vi "Autonomous Independent.vi"() -> ()   [LabVIEW 2016]
doc: "This VI is called when autonomous begins, and will automatically be terminated when autonomous ends. You can carry out timed or sensor driven robot movement independently without needing to return to the caller."
uses:
  <vilib>/Rock Robotics/Network Tables/NT Read Number.vi
  Global 2.vi
  Systems/Global 1.vi
panel:
  out "Waveform Graph":dbl[](graph)=[24.733139233474137]
  out "Numeric":i32=72
  out "Gyro":dbl=0.0502646432904
  in  "Oscillate effort":dbl=0.25 format="%#_13g"
  out "Auto Mode":dbl=2.0
  in  "Auton_Modes":T1(array[cluster])=[{"Actions"=[{"Effort"=0.55, "Duration"=3.5, "Action"=enum."Vision Correction", "Encoder"=0.0, "Condition"=FALSE}, {"Effort"=0.0, "Duration"=0.0, "Action"=enum."Nothing", "Encoder"=0.0, "Condition"=FALSE}]}, {"Actions"=[{"Effort"=0.53, "Duration"=1.0, "Action"=enum."Shoot", "Encoder"=6.462, "Condition"=TRUE}, {"Effort"=0.0, "Duration"=3.0, "Action"=enum."Index", "Encoder"=0.0, "Condition"=FALSE}, {"Effort"=0.3, "Duration"=2.0, "Action"=enum."Turn", "Encoder"=38.0, "Condition"=FALSE}, {"Effort"=0.3, "Duration"=5.0, "Action"=enum."Drive", "Encoder"=0.0, "Condition"=TRUE}, {"Effort"=0.25, "Duration"=0.0, "Action"=enum."Nothing", "Encoder"=57.0, "Condition"=FALSE}, {"Effort"=-0.25, "Duration"=0.0, "Action"=enum."Nothing", "Encoder"=0.0, "Condition"=FALSE}, {"Effort"=1.0, "Duration"=0.0, "Action"=enum."Nothing", "Encoder"=0.0, "Condition"=FALSE}, {"Effort"=0.25, "Duration"=0.0, "Action"=enum."Nothing", "Encoder"=0.0, "Condition"=FALSE}]}, {"Actions"=[{"Effort"=0.0, "Duration"=0.1, "Action"=enum."Drive Encoder Reset", "Encoder"=0.0, "Condition"=FALSE}, {"Effort"=0.0, "Duration"=0.1, "Action"=enum."Gyro Reset", "Encoder"=0.0, "Condition"=FALSE}, {"Effort"=0.3, "Duration"=2.5, "Action"=enum."Drive", "Encoder"=50.0, "Condition"=FALSE}, {"Effort"=1.0, "Duration"=1.0, "Action"=enum."Gear0", "Encoder"=0.0, "Condition"=FALSE}, {"Effort"=1.0, "Duration"=0.0, "Action"=enum."Nothing", "Encoder"=0.0, "Condition"=FALSE}, {"Effort"=1.0, "Duration"=0.5, "Action"=enum."Nothing", "Encoder"=0.0, "Condition"=FALSE}, {"Effort"=0.0, "Duration"=0.0, "Action"=enum."Drive Encoder Reset", "Encoder"=0.0, "Condition"=FALSE}, {"Effort"=0.3, "Duration"=0.5, "Action"=enum."Nothing", "Encoder"=10.0, "Condition"=FALSE}, {"Effort"=0.0, "Duration"=0.0, "Action"=enum."Nothing", "Encoder"=0.0, "Condition"=FALSE}, {"Effort"=-0.2, "Duration"=10000.0, "Action"=enum."Drive", "Encoder"=24.0, "Condition"=FALSE}, {"Effort"=0.0, "Duration"=0.0, "Action"=enum."Drive Encoder Reset", "Encoder"=0.0, "Condition"=FALSE}, {"Effort"=-0.25, "Duration"=0.0, "Action"=enum."Nothing", "Encoder"=12.0, "Condition"=FALSE}]}, {"Actions"=[{"Effort"=0.0, "Duration"=0.1, "Action"=enum."Drive Encoder Reset", "Encoder"=6.462, "Condition"=FALSE}, {"Effort"=0.0, "Duration"=0.1, "Action"=enum."Gyro Reset", "Encoder"=0.0, "Condition"=FALSE}, {"Effort"=-0.25, "Duration"=1.0, "Action"=enum."Drive", "Encoder"=6.462, "Condition"=FALSE}, {"Effort"=0.0, "Duration"=0.1, "Action"=enum."Gyro Reset", "Encoder"=0.0, "Condition"=FALSE}, {"Effort"=-0.25, "Duration"=0.0, "Action"=enum."Turn", "Encoder"=0.0, "Condition"=FALSE}, {"Effort"=-0.25, "Duration"=0.0, "Action"=enum."Drive", "Encoder"=7.5, "Condition"=FALSE}, {"Effort"=-1.0, "Duration"=0.0, "Action"=enum."Gear0", "Encoder"=0.0, "Condition"=FALSE}, {"Effort"=0.25, "Duration"=0.0, "Action"=enum."Drive", "Encoder"=3.0, "Condition"=FALSE}]}, {"Actions"=[{"Effort"=0.0, "Duration"=0.1, "Action"=enum."Drive Encoder Reset", "Encoder"=6.462, "Condition"=FALSE}, {"Effort"=0.0, "Duration"=0.1, "Action"=enum."Gyro Reset", "Encoder"=0.0, "Condition"=FALSE}, {"Effort"=-0.25, "Duration"=1.0, "Action"=enum."Drive", "Encoder"=6.462, "Condition"=FALSE}, {"Effort"=0.0, "Duration"=0.1, "Action"=enum."Gyro Reset", "Encoder"=0.0, "Condition"=FALSE}, {"Effort"=-0.25, "Duration"=0.0, "Action"=enum."Turn", "Encoder"=0.0, "Condition"=FALSE}, {"Effort"=-0.25, "Duration"=0.0, "Action"=enum."Drive", "Encoder"=7.5, "Condition"=FALSE}, {"Effort"=-1.0, "Duration"=0.0, "Action"=enum."Gear0", "Encoder"=0.0, "Condition"=FALSE}, {"Effort"=0.25, "Duration"=0.0, "Action"=enum."Drive", "Encoder"=3.0, "Condition"=FALSE}]}, {"Actions"=[{"Effort"=0.0, "Duration"=0.1, "Action"=enum."Drive Encoder Reset", "Encoder"=0.0, "Condition"=FALSE}, {"Effort"=0.0, "Duration"=0.1, "Action"=enum."Gyro Reset", "Encoder"=0.0, "Condition"=FALSE}, {"Effort"=0.25, "Duration"=1.0, "Action"=enum."Drive", "Encoder"=6.462, "Condition"=FALSE}, {"Effort"=1.0, "Duration"=0.1, "Action"=enum."Gyro Reset", "Encoder"=0.0, "Condition"=FALSE}, {"Effort"=0.25, "Duration"=0.0, "Action"=enum."Turn", "Encoder"=0.0, "Condition"=FALSE}, {"Effort"=0.25, "Duration"=0.0, "Action"=enum."Drive", "Encoder"=7.5, "Condition"=FALSE}, {"Effort"=1.0, "Duration"=0.0, "Action"=enum."Gear0", "Encoder"=0.0, "Condition"=FALSE}, {"Effort"=-0.25, "Duration"=0.0, "Action"=enum."Drive", "Encoder"=3.0, "Condition"=FALSE}]}, {"Actions"=[{"Effort"=0.0, "Duration"=0.1, "Action"=enum."Nothing", "Encoder"=0.0, "Condition"=FALSE}, {"Effort"=0.0, "Duration"=0.1, "Action"=enum."Gyro Reset", "Encoder"=0.0, "Condition"=FALSE}, {"Effort"=0.25, "Duration"=5.0, "Action"=enum."Drive", "Encoder"=60000.0, "Condition"=TRUE}, {"Effort"=0.75, "Duration"=1.0, "Action"=enum."Nothing", "Encoder"=0.0, "Condition"=FALSE}, {"Effort"=0.0, "Duration"=1.0, "Action"=enum."Nothing", "Encoder"=0.0, "Condition"=FALSE}, {"Effort"=0.0, "Duration"=0.0, "Action"=enum."Nothing", "Encoder"=0.0, "Condition"=FALSE}]}, {"Actions"=[{"Effort"=0.0, "Duration"=0.5, "Action"=enum."Drive Encoder Reset", "Encoder"=0.0, "Condition"=FALSE}, {"Effort"=0.55, "Duration"=4.25, "Action"=enum."Gyro Reset", "Encoder"=0.0, "Condition"=FALSE}, {"Effort"=-0.5, "Duration"=0.0, "Action"=enum."Drive", "Encoder"=46.0, "Condition"=FALSE}, {"Effort"=0.3, "Duration"=1.0, "Action"=enum."Nothing", "Encoder"=0.0, "Condition"=FALSE}, {"Effort"=0.3, "Duration"=2.0, "Action"=enum."Vision Correction", "Encoder"=76.6, "Condition"=FALSE}, {"Effort"=-0.25, "Duration"=1.0, "Action"=enum."Drive", "Encoder"=18.5, "Condition"=TRUE}, {"Effort"=1.0, "Duration"=0.0, "Action"=enum."Gear0", "Encoder"=0.0, "Condition"=FALSE}, {"Effort"=0.3, "Duration"=1.3, "Action"=enum."Drive", "Encoder"=30.0, "Condition"=TRUE}, {"Effort"=0.0, "Duration"=0.0, "Action"=enum."Nothing", "Encoder"=0.0, "Condition"=FALSE}, {"Effort"=0.03, "Duration"=0.0, "Action"=enum."Turn", "Encoder"=0.0, "Condition"=FALSE}, {"Effort"=0.0, "Duration"=0.0, "Action"=enum."Drive", "Encoder"=0.0, "Condition"=FALSE}]}, {"Actions"=[{"Effort"=0.0, "Duration"=0.0, "Action"=enum."Nothing", "Encoder"=0.0, "Condition"=FALSE}]}, {"Actions"=[{"Effort"=0.0, "Duration"=2.5, "Action"=enum."Shoot", "Encoder"=0.0, "Condition"=FALSE}, {"Effort"=0.0, "Duration"=5.0, "Action"=enum."Index", "Encoder"=0.0, "Condition"=FALSE}, {"Effort"=0.25, "Duration"=3.5, "Action"=enum."Nothing", "Encoder"=88.0, "Condition"=FALSE}, {"Effort"=1.0, "Duration"=1.0, "Action"=enum."Nothing", "Encoder"=0.0, "Condition"=FALSE}, {"Effort"=1.0, "Duration"=1.0, "Action"=enum."Nothing", "Encoder"=0.0, "Condition"=FALSE}, {"Effort"=1.0, "Duration"=0.5, "Action"=enum."Nothing", "Encoder"=0.0, "Condition"=FALSE}, {"Effort"=0.0, "Duration"=0.0, "Action"=enum."Nothing", "Encoder"=0.0, "Condition"=FALSE}, {"Effort"=-0.25, "Duration"=0.0, "Action"=enum."Nothing", "Encoder"=3.0, "Condition"=FALSE}, {"Effort"=0.0, "Duration"=0.0, "Action"=enum."Nothing", "Encoder"=0.0, "Condition"=FALSE}, {"Effort"=0.25, "Duration"=0.0, "Action"=enum."Nothing", "Encoder"=24.0, "Condition"=FALSE}, {"Effort"=0.0, "Duration"=0.0, "Action"=enum."Nothing", "Encoder"=0.0, "Condition"=FALSE}, {"Effort"=-0.25, "Duration"=0.0, "Action"=enum."Nothing", "Encoder"=12.0, "Condition"=FALSE}]}, {"Actions"=[{"Effort"=0.0, "Duration"=0.1, "Action"=enum."Drive Encoder Reset", "Encoder"=0.0, "Condition"=FALSE}, {"Effort"=0.0, "Duration"=1.0, "Action"=enum."Gyro Reset", "Encoder"=0.0, "Condition"=FALSE}, {"Effort"=0.3, "Duration"=1.4, "Action"=enum."Drive", "Encoder"=88.0, "Condition"=TRUE}, {"Effort"=0.3, "Duration"=4.0, "Action"=enum."Turn", "Encoder"=2.0, "Condition"=FALSE}, {"Effort"=1.0, "Duration"=1.0, "Action"=enum."Nothing", "Encoder"=0.0, "Condition"=FALSE}, {"Effort"=1.0, "Duration"=0.5, "Action"=enum."Nothing", "Encoder"=0.0, "Condition"=FALSE}, {"Effort"=0.0, "Duration"=0.0, "Action"=enum."Nothing", "Encoder"=0.0, "Condition"=FALSE}, {"Effort"=-0.25, "Duration"=0.0, "Action"=enum."Nothing", "Encoder"=3.0, "Condition"=FALSE}, {"Effort"=0.0, "Duration"=0.0, "Action"=enum."Nothing", "Encoder"=0.0, "Condition"=FALSE}, {"Effort"=0.25, "Duration"=0.0, "Action"=enum."Nothing", "Encoder"=24.0, "Condition"=FALSE}, {"Effort"=0.0, "Duration"=0.0, "Action"=enum."Nothing", "Encoder"=0.0, "Condition"=FALSE}, {"Effort"=-0.25, "Duration"=0.0, "Action"=enum."Nothing", "Encoder"=12.0, "Condition"=FALSE}]}, {"Actions"=[{"Effort"=0.0, "Duration"=1.0, "Action"=enum."Drive Encoder Reset", "Encoder"=0.0, "Condition"=FALSE}, {"Effort"=0.0, "Duration"=1.0, "Action"=enum."Shoot", "Encoder"=0.0, "Condition"=FALSE}, {"Effort"=0.25, "Duration"=5.0, "Action"=enum."Index", "Encoder"=88.0, "Condition"=FALSE}, {"Effort"=1.0, "Duration"=1.0, "Action"=enum."Nothing", "Encoder"=0.0, "Condition"=FALSE}, {"Effort"=1.0, "Duration"=1.0, "Action"=enum."Nothing", "Encoder"=0.0, "Condition"=FALSE}, {"Effort"=1.0, "Duration"=0.5, "Action"=enum."Nothing", "Encoder"=0.0, "Condition"=FALSE}, {"Effort"=0.0, "Duration"=0.0, "Action"=enum."Nothing", "Encoder"=0.0, "Condition"=FALSE}, {"Effort"=-0.25, "Duration"=0.0, "Action"=enum."Nothing", "Encoder"=3.0, "Condition"=FALSE}, {"Effort"=0.0, "Duration"=0.0, "Action"=enum."Nothing", "Encoder"=0.0, "Condition"=FALSE}, {"Effort"=0.25, "Duration"=0.0, "Action"=enum."Nothing", "Encoder"=24.0, "Condition"=FALSE}, {"Effort"=0.0, "Duration"=0.0, "Action"=enum."Nothing", "Encoder"=0.0, "Condition"=FALSE}, {"Effort"=-0.25, "Duration"=0.0, "Action"=enum."Nothing", "Encoder"=12.0, "Condition"=FALSE}]}, {"Actions"=[{"Effort"=0.0, "Duration"=0.1, "Action"=enum."Drive Encoder Reset", "Encoder"=0.0, "Condition"=FALSE}, {"Effort"=0.0, "Duration"=1.0, "Action"=enum."Gyro Reset", "Encoder"=0.0, "Condition"=FALSE}, {"Effort"=0.3, "Duration"=1.4, "Action"=enum."Drive", "Encoder"=88.0, "Condition"=TRUE}, {"Effort"=0.3, "Duration"=4.0, "Action"=enum."Turn", "Encoder"=0.0, "Condition"=FALSE}, {"Effort"=1.0, "Duration"=1.0, "Action"=enum."Nothing", "Encoder"=0.0, "Condition"=FALSE}, {"Effort"=1.0, "Duration"=0.5, "Action"=enum."Nothing", "Encoder"=0.0, "Condition"=FALSE}, {"Effort"=0.0, "Duration"=0.0, "Action"=enum."Nothing", "Encoder"=0.0, "Condition"=FALSE}, {"Effort"=0.3, "Duration"=0.5, "Action"=enum."Nothing", "Encoder"=24.0, "Condition"=TRUE}, {"Effort"=0.0, "Duration"=0.0, "Action"=enum."Nothing", "Encoder"=0.0, "Condition"=FALSE}, {"Effort"=-0.2, "Duration"=2.0, "Action"=enum."Nothing", "Encoder"=24.0, "Condition"=TRUE}, {"Effort"=0.0, "Duration"=0.0, "Action"=enum."Nothing", "Encoder"=0.0, "Condition"=FALSE}, {"Effort"=-0.25, "Duration"=0.0, "Action"=enum."Nothing", "Encoder"=12.0, "Condition"=FALSE}]}]
  # "Nothing"
  # "Boiler Right Right side gear"
  # "Middle Gear"
  # "Boiler Right Left Side Gear"
  # "Boiler Left RightSide Gear"
  # "Boiler Left Left Side Gear"
  # "Drive"
  # "Vision Correction"
  # "Hopper"
  # "10 ball"
  # "Farside"
  # "Boilerside-10 ball"
  # "Auto 5"
  # "Auto 6"
  # "Auto 6"
  # "Auto 7"
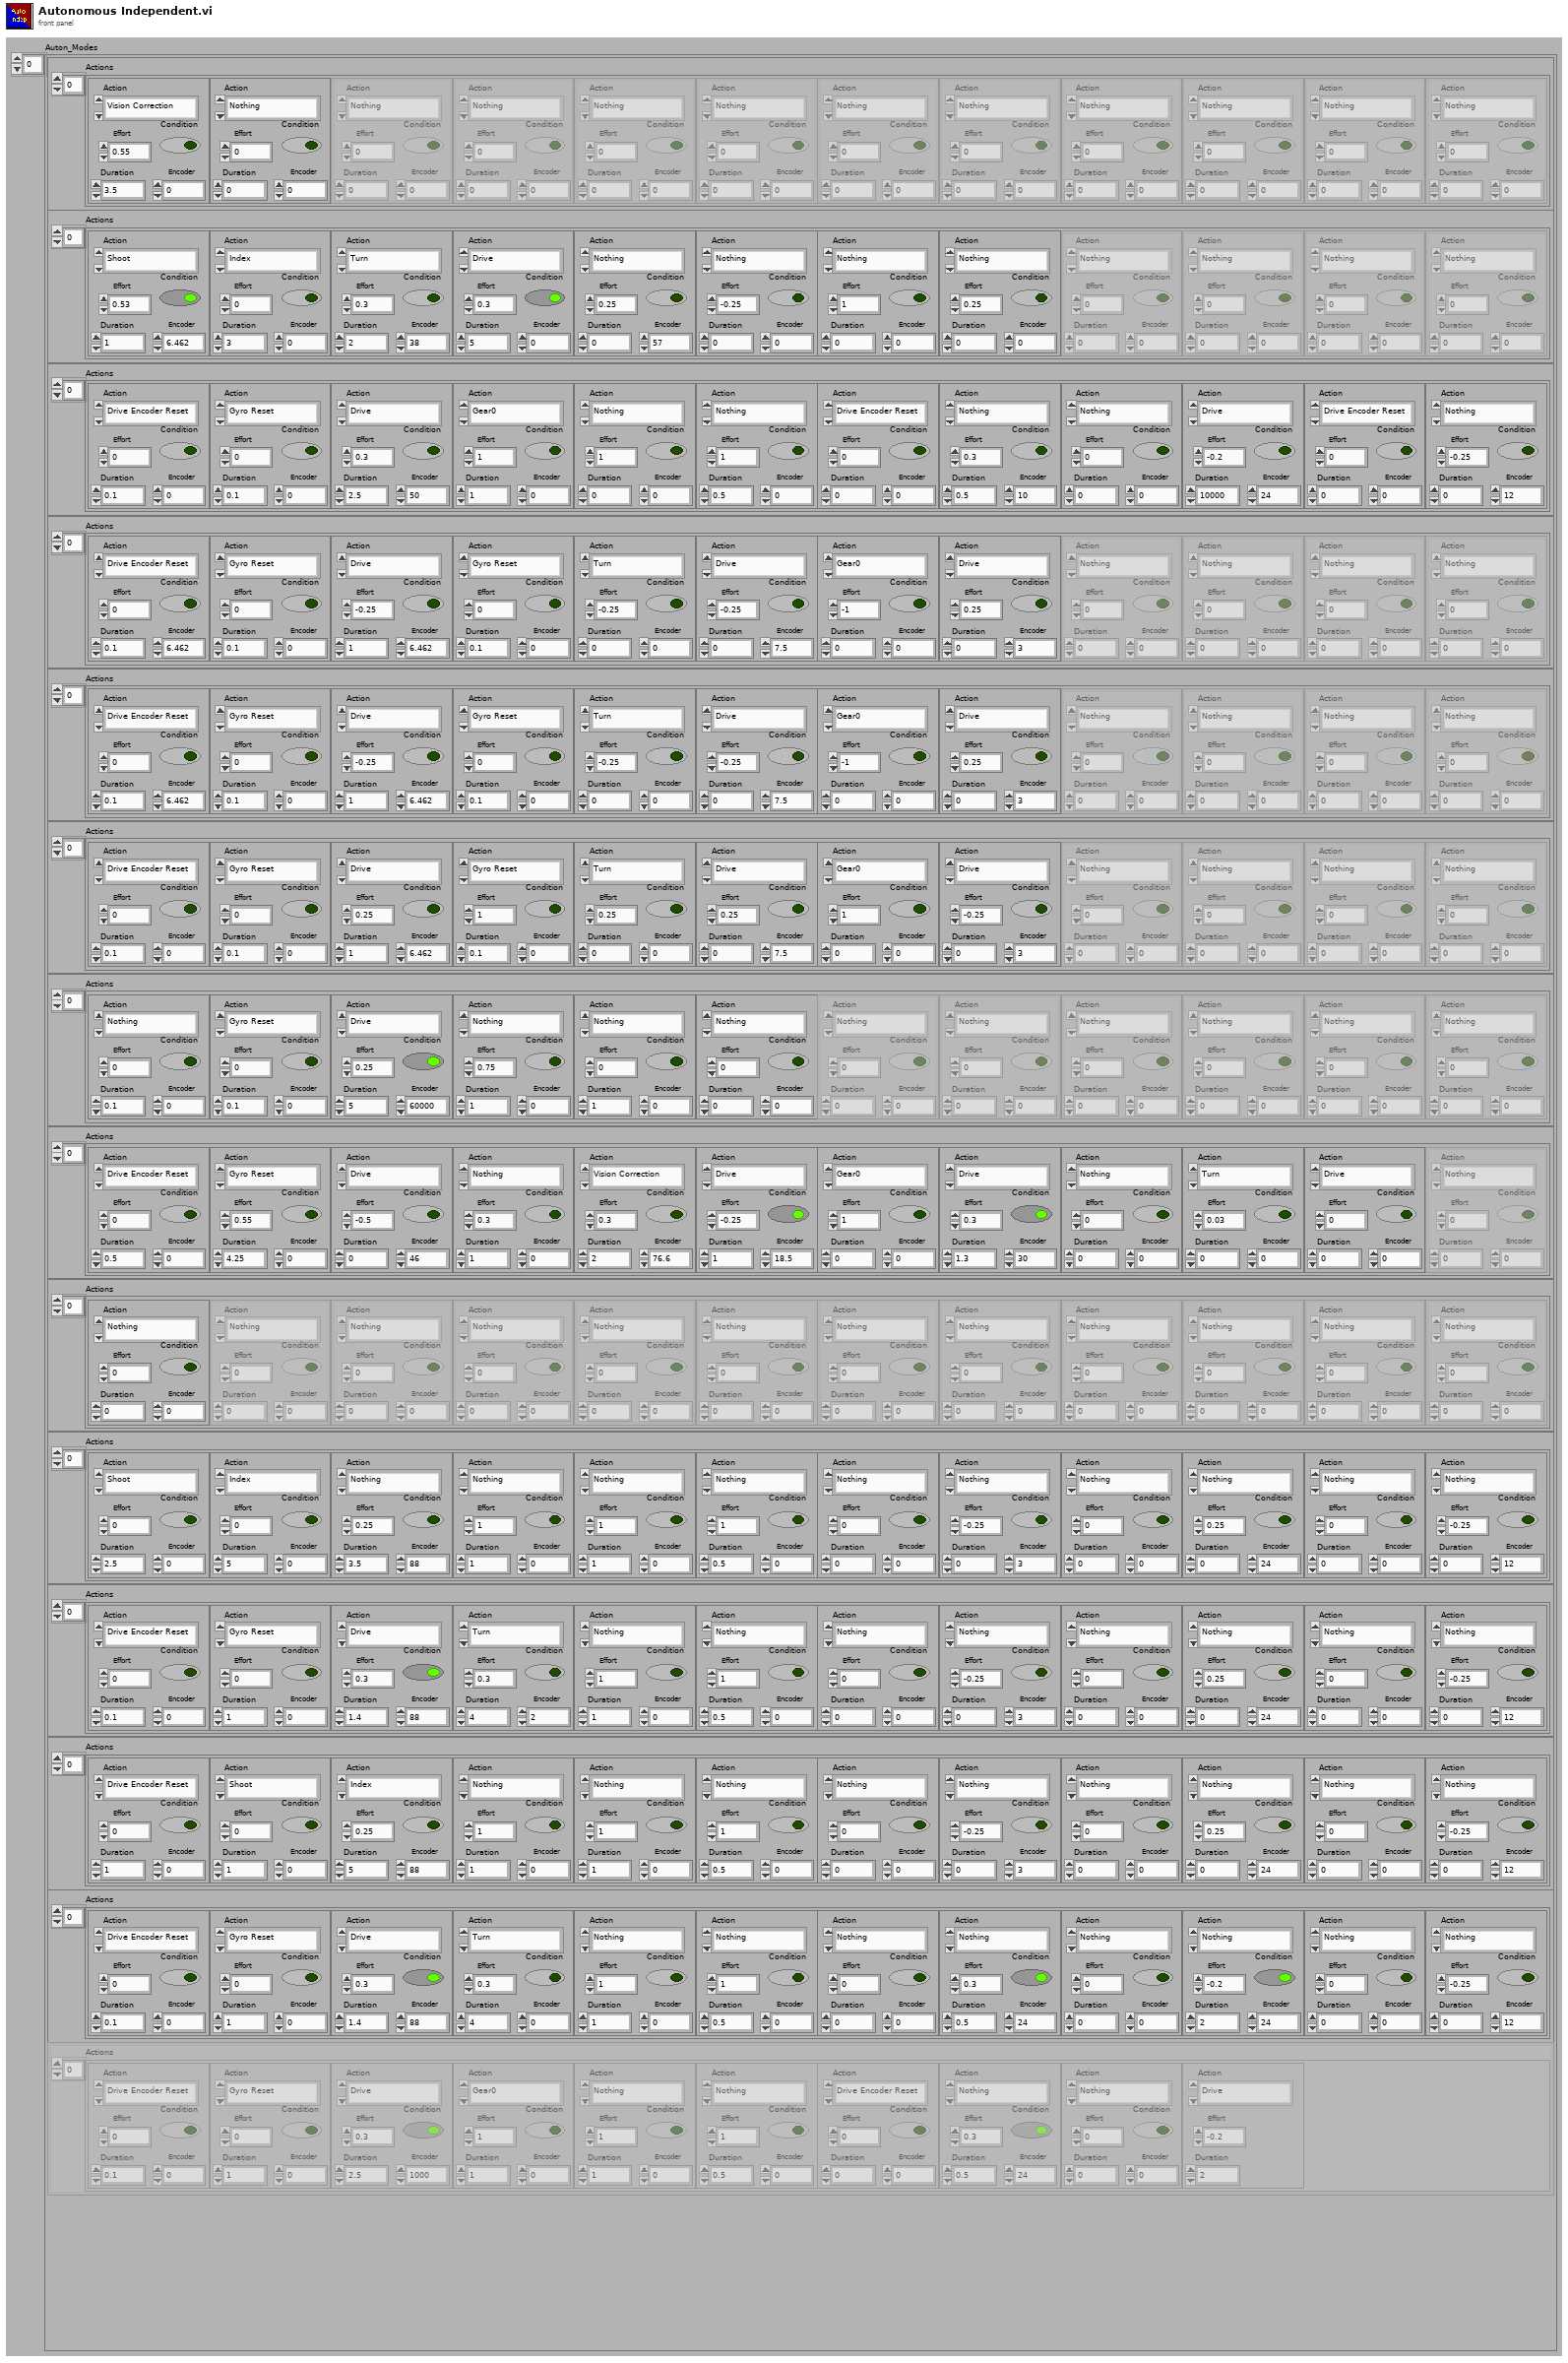
[diagram p1: front panel]
types:
  T1 = cluster{"Actions":cluster{"Effort":dbl, "Duration":dbl, "Action":enum16{"Nothing", "Drive", "Vision Correction", "Turn", "Gear0", "Gear1", "Climb", "Intake", "Index", "Shoot", "Test", "Drive Encoder Reset", "Gyro Reset"}, "Encoder":dbl, "Condition":bool}[]}[]
  T2 = cluster{"Actions":cluster{"Effort":dbl, "Duration":dbl, "Action":enum16{"Nothing", "Drive", "Vision Correction", "Turn", "Gear0", "Gear1", "Climb", "Intake", "Index", "Shoot", "Test", "Drive Encoder Reset", "Gyro Reset"}, "Encoder":dbl, "Condition":bool}[]}
  T3 = cluster{"Effort":dbl, "Duration":dbl, "Action":enum16{"Nothing", "Drive", "Vision Correction", "Turn", "Gear0", "Gear1", "Climb", "Intake", "Index", "Shoot", "Test", "Drive Encoder Reset", "Gyro Reset"}, "Encoder":dbl, "Condition":bool}[]
  T4 = enum16{"Nothing", "Drive", "Vision Correction", "Turn", "Gear0", "Gear1", "Climb", "Intake", "Index", "Shoot", "Test", "Drive Encoder Reset", "Gyro Reset"}
  T5 = typedef "WPI_MotorControlDeviceRef.ctl" = cluster{"DeviceStatus":errorcluster, "Type":T6, "PWM":cluster{"PWM Channel":T7, "DeadBand":T8}, "CAN":cluster{"Device Number":u8, "SetOutput VI Ref":variant, "GetOutput VI Ref":variant, "Enable VI Ref":variant, "Disable VI Ref":variant, "Data":variant}, "Invert":bool}
  T6 = typedef "WPI_MotorControlType.ctl" = enum16{"PWM", "CAN"}
  T7 = typedef "FPGA_DIOPWMChannel.ctl" = enum8{"PWM 0", "PWM 1", "PWM 2", "PWM 3", "PWM 4", "PWM 5", "PWM 6", "PWM 7", "PWM 8", "PWM 9", "PWM MXP 0", "PWM MXP 1", "PWM MXP 2", "PWM MXP 3", "PWM MXP 4", "PWM MXP 5", "PWM MXP 6", "PWM MXP 7", "PWM MXP 8", "PWM MXP 9", "Invalid"}
  T8 = typedef "WPI_PWMDeadband.ctl" = cluster{"Name":string, "maxPositivePwm":i32, "minPositivePwm":i32, "centerPwm":i32, "maxNegativePwm":i32, "minNegativePwm":i32, "angularRange":u16}
  T9 = typedef "WPI_CANTalonSRX_GlobalStatus.ctl" = cluster{"Applied Throttle":dbl, "Module Enabled":bool, "CAN Error":errorcluster, "Closed Loop Error":dbl, "Forward Limit Switch Closed":bool, "Reverse Limit Switch Closed":bool, "Sensor Position":dbl, "Sensor Velocity":dbl, "Current":dbl, "Sticky Fault - Over Temp":bool, "Sticky Fault - Under Voltage":bool, "Sticky Fault - Forward Limit":bool, "Sticky Fault - Reverse Limit":bool, "Sticky Fault - Forward Soft Limit":bool, "Sticky Fault - Reverse Soft Limit":bool, "Brake is Enabled":bool, "Encoder Position":dbl, "Encoder Velocity":dbl, "Encoder Index Count":dbl, "Encoder A Pin State":bool, "Encoder B Pin State":bool, "Encoder Index Pin State":bool, "Analog In":dbl, "Analog In Velocity":dbl, "Temperature (C)":dbl, "Battery Voltage":dbl, "Control 5 Is Supported":bool, "Current Profile Slot Select":dbl, "Pos Div 8":bool, "Vel Div 4":bool, "Pulse Width Position":i32, "Pulse Width Velocity":i32, "Pulse Width Rise To Rise (us)":i32, "Pulse Width Rise To Fall (us)":i32, "Mot Prof Active Is Under Run":bool, "Mot Prof Active Has Under Run":bool, "Mot Prof Active Is Last":bool, "Mot Prof Active Velocity Only":bool, "Mot Prof Active Is Valid":bool, "Mot Prof Buffer Is Full":bool, "Mot Prof Active Profile Slot Select":i32, "Mot Prof NextID":i32, "Mot Prof Count":i32, "Mot Prof Active Velocity":dbl, "Mot Prof Active Position":dbl, "Mot Prof Output Enable":i32}
  T10 = typedef "WPI_GyroDevRef.ctl" = cluster{"DevStatus":errorcluster, "Analog Channel":T11, "Offset":dbl, "Gain (VoltsPerDegree/Second)":dbl, "Gyro Type":enum16{"Analog", "XRS450"}, "Handle":i32, "SPI Bus":T12, "Device Found":bool, "Sample Rate":dbl, "Calibrate On Open":bool}
  T11 = typedef "FPGA_AIChannel.ctl" = enum8{"AI 0", "AI 1", "AI 2", "AI 3", "AI MXP 0", "AI MXP 1", "AI MXP 2", "AI MXP 3", "Invalid"}
  T12 = typedef "spi_bus.ctl" = enum16{"SPI On-Board, CS0", "SPI On-Board, CS1", "SPI On-Board, CS2", "SPI On-Board, CS3", "SPI MXP", "Invalid"}
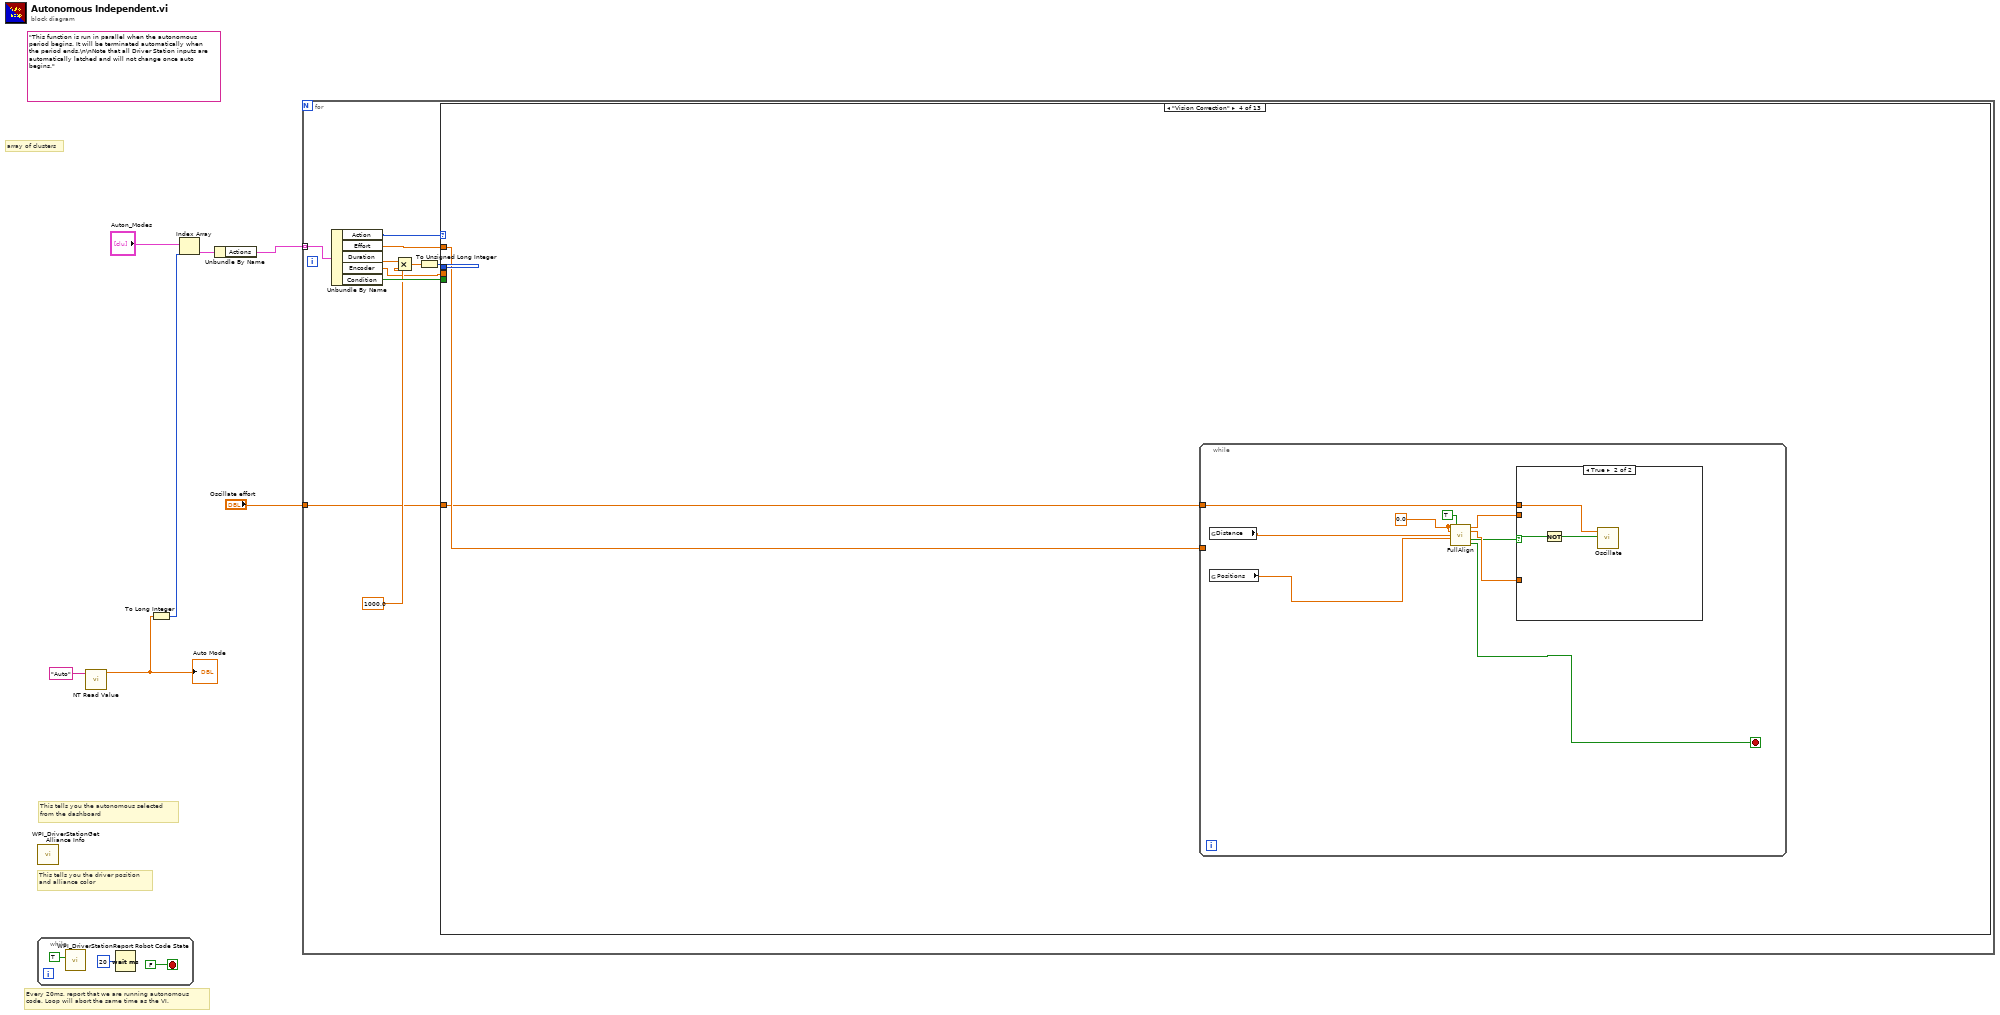
[diagram p0: block diagram]
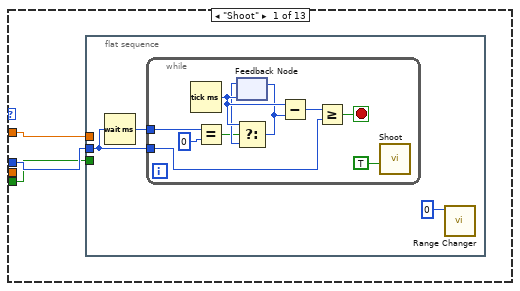
[diagram p2: hidden frame]
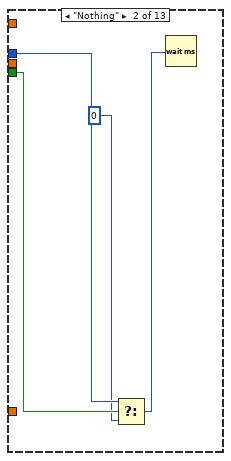
[diagram p3: hidden frame]
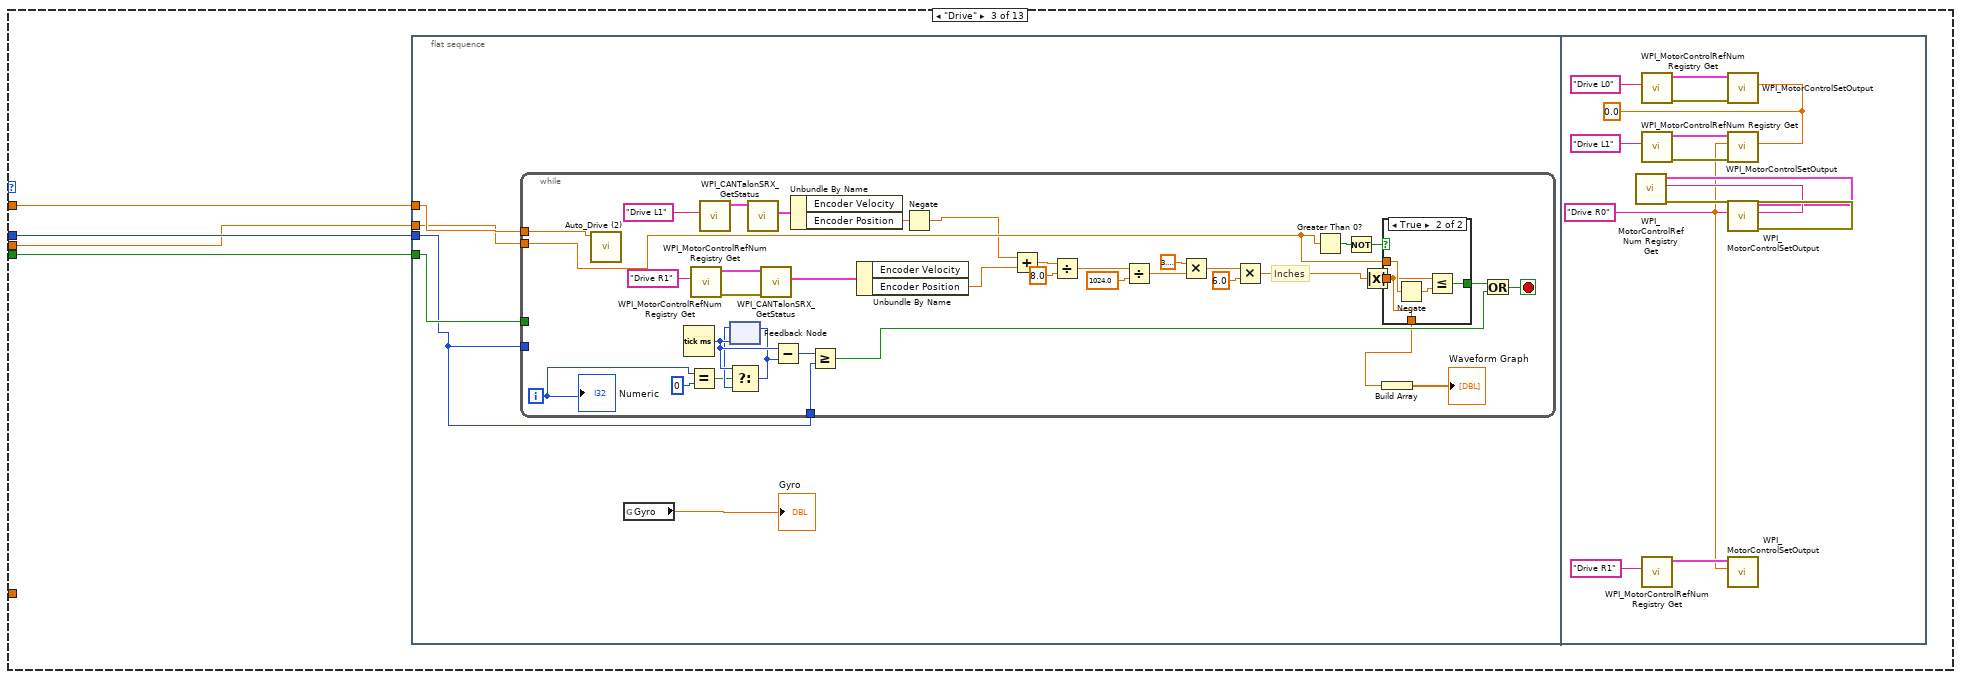
[diagram p4: hidden frame]
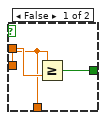
[diagram p5: hidden frame]
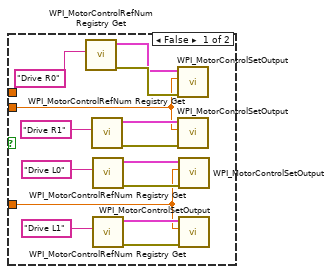
[diagram p6: hidden frame]
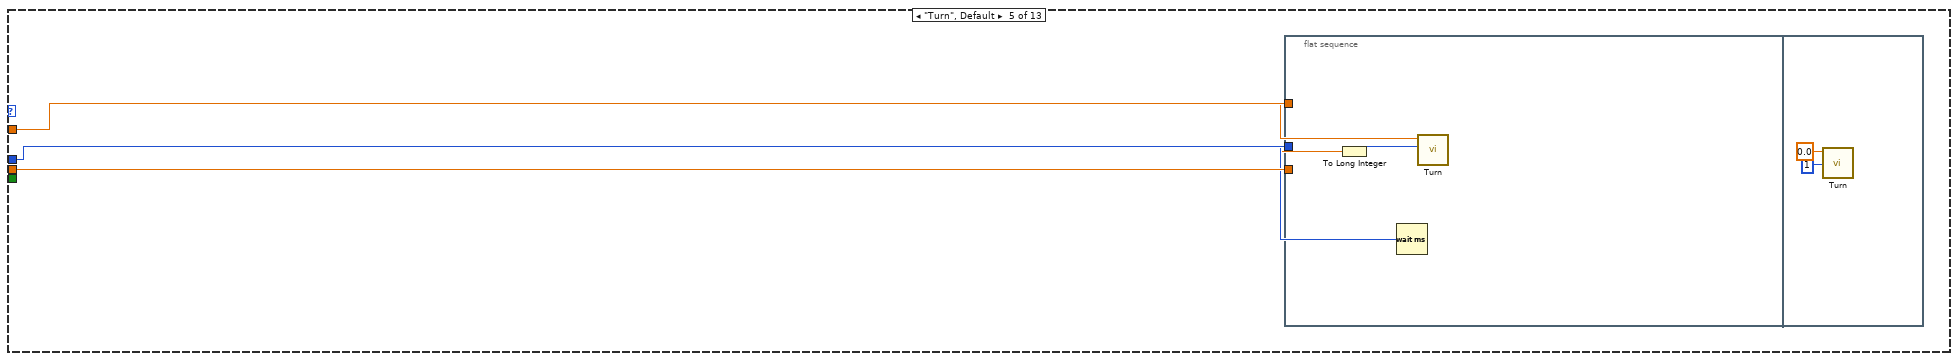
[diagram p7: hidden frame]
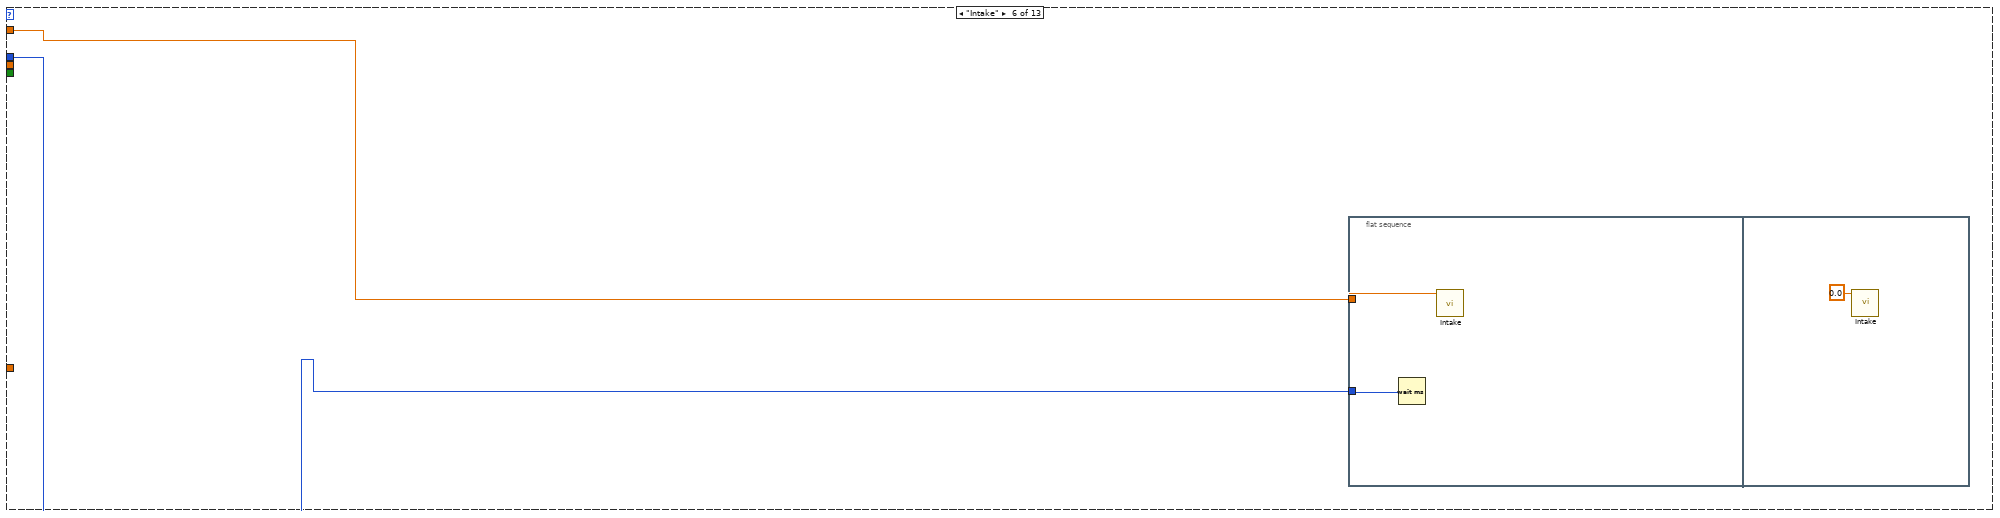
[diagram p8: hidden frame]
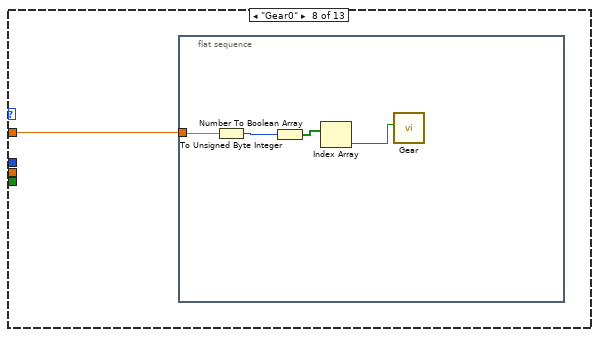
[diagram p10: hidden frame]
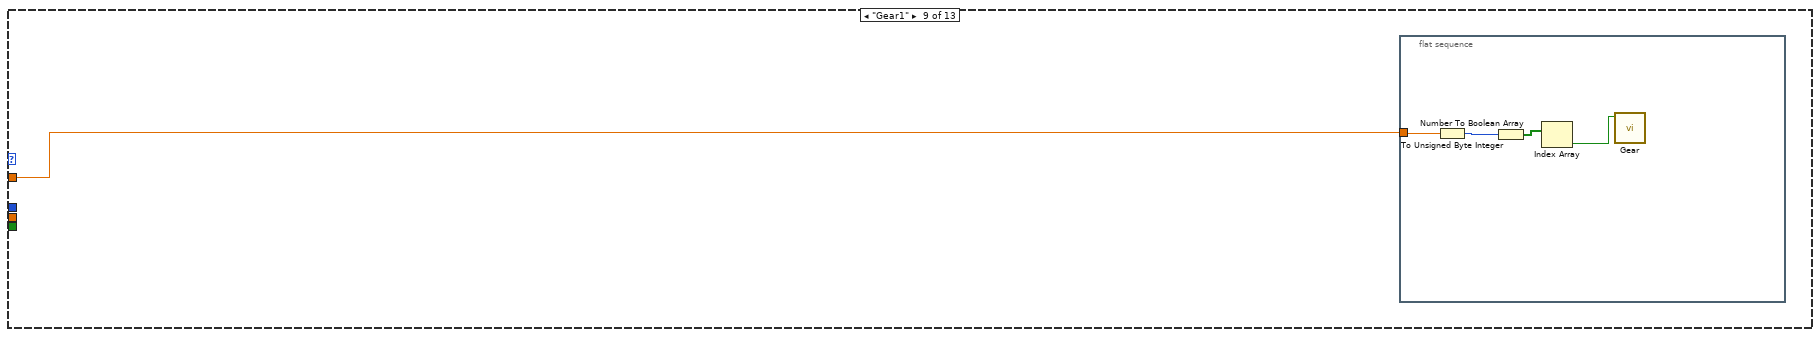
[diagram p11: hidden frame]
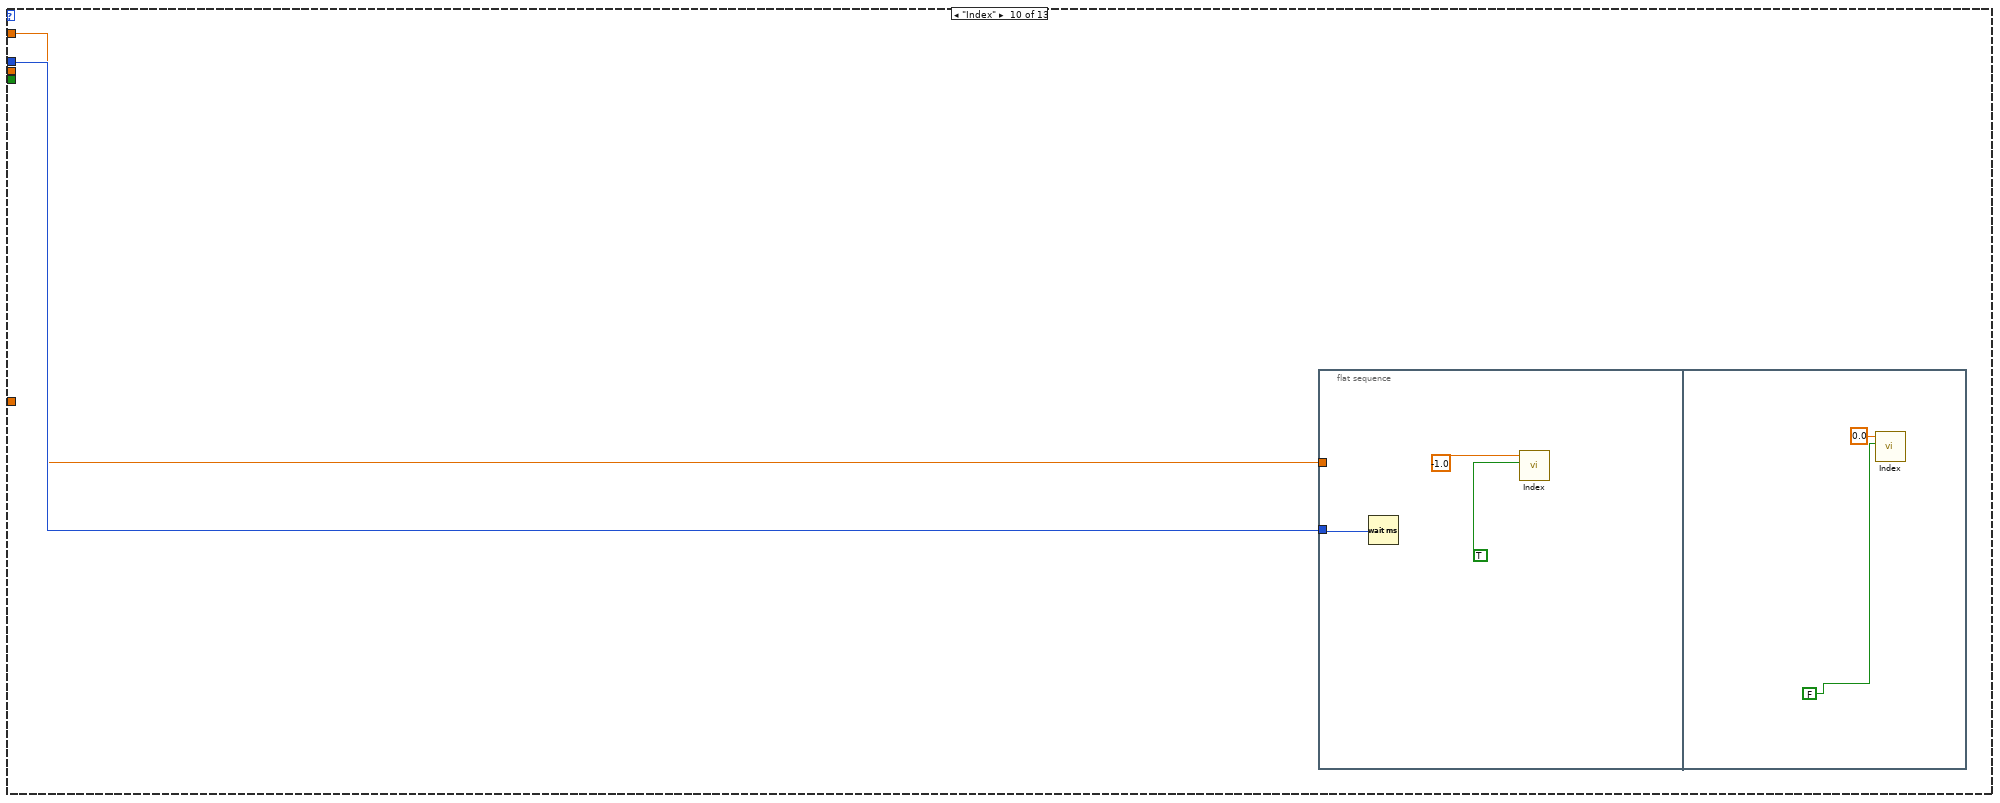
[diagram p12: hidden frame]
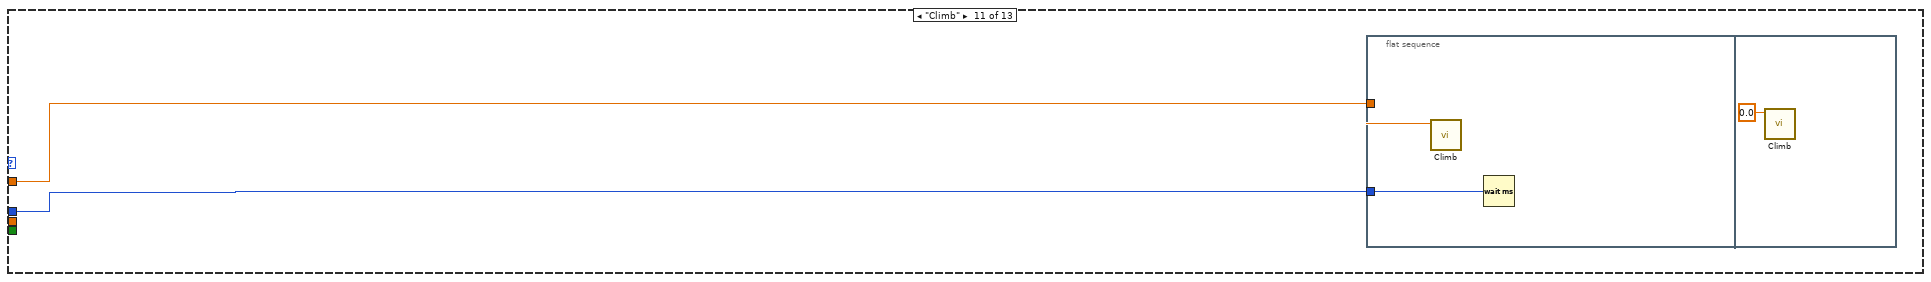
[diagram p13: hidden frame]
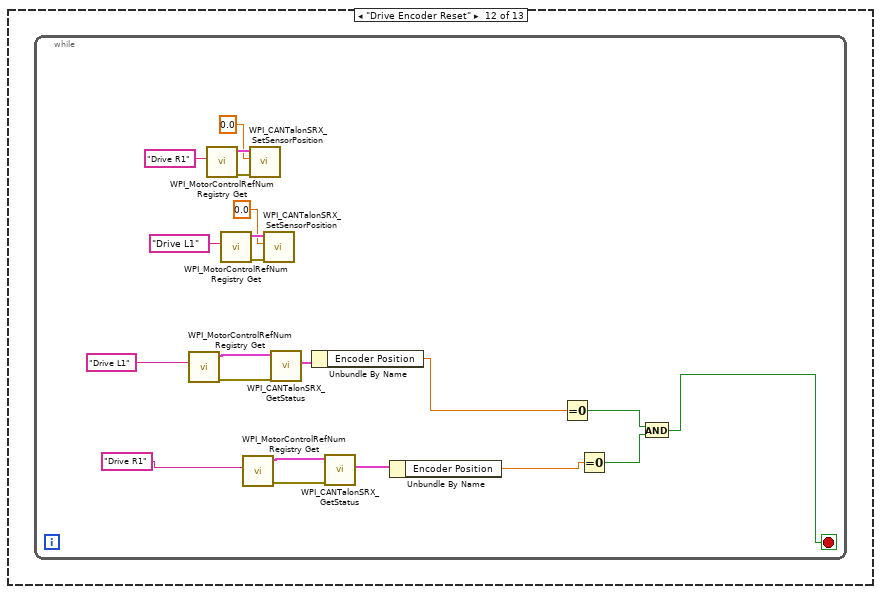
[diagram p14: hidden frame]
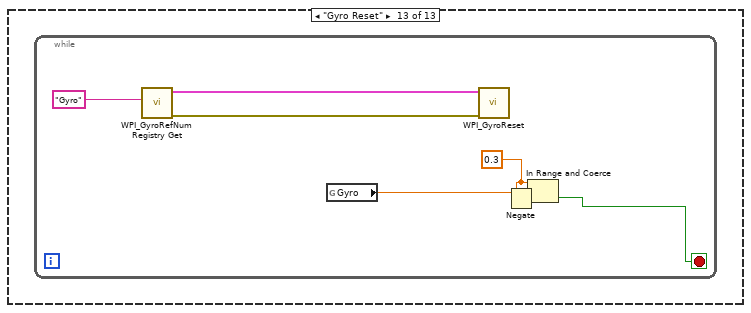
[diagram p15: hidden frame]
diagram:
  (unwired) "This function is run in parallel when the autonomous period begins. It will be terminated automatically when the period ends.\n\nNote that all Driver Station inputs are automatically latched and will not change once auto begins."
  # "This tells you the autonomous selected\nfrom the dashboard"
  # "array of clusters"
  # "Every 20ms, report that we are running autonomous\ncode. Loop will abort the same time as the VI."
  # "This tells you the driver position\nand alliance color"
  n1 = while {
    stop <- FALSE stop-if-true
    n2 = call <vilib>:"WPI_DriverStationReport Robot Code State.vi"("Autonomous"=TRUE) -> ()  [unwired: 10 in, 1 out]
    n3 = Wait (ms)(milliseconds to wait=u32 20) -> ()  [unwired: 1 out]
  }
  n4 = call <vilib>:"WPI_DriverStationGet Alliance Info.vi"() -> ()  [unwired: 12 out]
  n5 = call-poly <vilib>:"NT Read Value.vi"("Name"="Auto") -> ("Numeric"=w2:dbl)  [unwired: 9 in, 1 out]
  "Auto Mode" <- w2
  n6 = To Long Integer(number=w2) -> (32bit integer=w4:i32)
  n7 = Index Array(array="Auton_Modes", index=w4) -> (element=w6:T2)
  n8 = Unbundle By Name(w6) -> ("Actions"=w7:T3)
  n9 = for {
    tunnel: w7 -> [w20] mode=indexing
    tunnel: "Oscillate effort" -> [w12]
    n10 = Unbundle By Name(w20) -> ("Action"=w11:T4, "Effort"=w19:dbl, "Duration"=w18:dbl, "Encoder"=w13:dbl, "Condition"=w15:bool)
    n11 = Multiply(x=w18, y=1000.0) -> (x*y=w17:dbl)
    n12 = To Unsigned Long Integer(number=w17) -> (unsigned 32bit integer=w16:u32)
    n13 = case shown="\"Vision Correction\"" w11 {
      tunnel: w19 -> [w23 _ w44 w107 w136 w144 _ w148 w153 w158 w166 _ _]
      tunnel: w16 -> [w22 w39 w43 _ w135 w143 _ _ _ w159 w165 _ _]
      tunnel: w15 -> [w21 w40 w42 _ _ _ _ _ _ _ _ _ _]
      tunnel: w13 -> [_ _ w41 _ w134 _ _ _ _ _ _ _ _]
      tunnel: w12 -> [_ _ _ w106 _ _ _ _ _ _ _ _ _]
      frame "Shoot" {
        n14 = flat-sequence {
          tunnel: w23 -> [_]
          tunnel: w22 -> [w24]
          tunnel: w21 -> [_]
          frame #0 {
            n15 = Wait (ms)(milliseconds to wait=w24) -> (millisecond timer value=w25:u32)
            n16 = while {
              tunnel: w25 -> [w28]
              tunnel: w24 -> [w27]
              stop <- w29 stop-if-true
              n17 = Tick Count (ms)() -> (millisecond timer value=w35:u32)
              n18 = Equal?(x=w28, y=0) -> (x = y?=w33:bool)
              n19 = feedback #1(w35) -> (w34:u32)
              n20 = Select(t=w35, s=w33, f=w34) -> (s? t:f=w31:u32)
              n21 = feedback-in #1(w31) -> ()
              n22 = Subtract(x=w35, y=w31) -> (x-y=w30:u32)
              n23 = Greater Or Equal?(x=w30, y=w27) -> (x >= y?=w29:bool)
              n24 = call "Shoot.vi"("Shoot"=TRUE) -> ()  [unwired: 10 in]
            }
            n25 = call "Range Changer.vi"("POV"=i16 0) -> ()  [unwired: 10 in, 1 out]
          }
        }
      }
      frame "Nothing" {
        n26 = Select(t=w39, s=w40, f=u32 0) -> (s? t:f=w37:u32)
        n27 = Wait (ms)(milliseconds to wait=w37) -> ()  [unwired: 1 out]
      }
      frame "Drive" {
        n28 = flat-sequence {
          tunnel: w44 -> [w49]
          tunnel: w43 -> [w45]
          tunnel: w42 -> [w47]
          tunnel: w41 -> [w48]
          frame #0 {
            n29 = while {
              tunnel: w49 -> [w86]
              tunnel: w48 -> [w73]
              tunnel: w47 -> [_]
              tunnel: w45 -> [_]
              tunnel: w45 -> [w66]
              i -> [w64]
              stop <- w74 stop-if-true
              # "Inches"
              n30 = call "Auto_Drive (2).vi"("Drive Effort"=w86) -> ()  [unwired: 11 in]
              n31 = Tick Count (ms)() -> (millisecond timer value=w72:u32)
              n32 = Equal?(x=w64, y=0) -> (x = y?=w70:bool)
              n33 = call <vilib>:"WPI_MotorControlRefNum Registry Get.vi"("refnum name"="Drive R1") -> ("error out"=w61:errorcluster, "MotorControlDevRef"=w60:T5)  [unwired: 9 in]
              n34 = call <vilib>:"WPI_MotorControlRefNum Registry Get.vi"("refnum name"="Drive L1") -> ("MotorControlDevRef"=w58:T5)  [unwired: 9 in, 1 out]
              n35 = feedback #2(w72) -> (w71:u32)
              n36 = Select(t=w72, s=w70, f=w71) -> (s? t:f=w68:u32)
              n37 = feedback-in #2(w68) -> ()
              n38 = call <vilib>:"WPI_CANTalonSRX_GetStatus.vi"("CAN Talon SRX Ref"=w58) -> ("Talon SRX Status"=w57:T9)  [unwired: 8 in, 2 out]
              n39 = call <vilib>:"WPI_CANTalonSRX_GetStatus.vi"("error in (no error)"=w61, "CAN Talon SRX Ref"=w60) -> ("Talon SRX Status"=w62:T9)  [unwired: 7 in, 2 out]
              n40 = Subtract(x=w72, y=w68) -> (x-y=w67:u32)
              n41 = Unbundle By Name(w57) -> ("Encoder Position"=w56:dbl)  [unwired: 1 out]
              n42 = Greater Or Equal?(x=w67, y=w66) -> (x >= y?=w65:bool)
              n43 = Unbundle By Name(w62) -> ("Encoder Position"=w54:dbl)  [unwired: 1 out]
              n44 = Negate(x=w56) -> (-x=w53:dbl)
              n45 = Add(x=w53, y=w54) -> (x+y=w85:dbl)
              n46 = Divide(x=w85, y=8.0) -> (x/y=w83:dbl)
              n47 = Divide(x=w83, y=1024.0) -> (x/y=w81:dbl)
              n48 = Multiply(x=3.141592653589793, y=w81) -> (x*y=w79:dbl)
              n49 = Multiply(x=w79, y=6.0) -> (x*y=w50:dbl)
              n50 = Greater Than 0?(x=w73) -> (x > 0?=w77:bool)
              n51 = Not(x=w77) -> (.not. x?=w75:bool)
              n52 = Absolute Value(x=w50) -> (abs(x)=w55:dbl)
              n53 = case shown="True" w75 {
                tunnel: [w89 w93] -> w76
                tunnel: w55 -> [w87 w90]
                tunnel: w73 -> [w88 w91]
                tunnel: [w87 w90] -> w52
                frame False {
                  n54 = Greater Or Equal?(x=w87, y=w88) -> (x >= y?=w89:bool)
                }
                frame True {
                  n55 = Negate(x=w91) -> (-x=w92:dbl)
                  n56 = Less Or Equal?(x=w90, y=w92) -> (x <= y?=w93:bool)
                }
              }
              n57 = Build Array(w52) -> (→"Waveform Graph":dbl[])
              n58 = Or(x=w76, y=w65) -> (x .or. y?=w74:bool)
              "Numeric" <- w64
            }
            n59 = global read "Global 2.vi" "Gyro"() -> (→"Gyro":dbl)
          }
          frame #1 {
            w94 = 0.0 ("Drive L")
            n60 = call <vilib>:"WPI_MotorControlRefNum Registry Get.vi"("refnum name"="Drive R0") -> ("error out"=w99:errorcluster, "MotorControlDevRef"=w95:T5)  [unwired: 9 in]
            n61 = call <vilib>:"WPI_MotorControlRefNum Registry Get.vi"("refnum name"="Drive L0") -> ("error out"=w100:errorcluster, "MotorControlDevRef"=w101:T5)  [unwired: 9 in]
            n62 = call <vilib>:"WPI_MotorControlRefNum Registry Get.vi"("refnum name"="Drive L1") -> ("error out"=w104:errorcluster, "MotorControlDevRef"=w103:T5)  [unwired: 9 in]
            n63 = call <vilib>:"WPI_MotorControlRefNum Registry Get.vi"("refnum name"="Drive R1") -> ("MotorControlDevRef"=w97:T5)  [unwired: 9 in, 1 out]
            n64 = call <vilib>:"WPI_MotorControlSetOutput.vi"("error in (no error)"=w100, "Output"=w94, "MotorControlDevRef"=w101) -> ()  [unwired: 6 in, 3 out]
            n65 = call <vilib>:"WPI_MotorControlSetOutput.vi"("error in (no error)"=w104, "Output"=w94, "MotorControlDevRef"=w103) -> ()  [unwired: 6 in, 3 out]
            n66 = call <vilib>:"WPI_MotorControlSetOutput.vi"("error in (no error)"=w99, "Output"=w94, "MotorControlDevRef"=w95) -> ()  [unwired: 6 in, 3 out]
            n67 = call <vilib>:"WPI_MotorControlSetOutput.vi"("Output"=w94, "MotorControlDevRef"=w97) -> ()  [unwired: 7 in, 3 out]
          }
        }
      }
      frame "Vision Correction" {
        n68 = while {
          tunnel: w107 -> [_]
          tunnel: w106 -> [w110]
          stop <- w111 stop-if-true
          w114 = 0.0
          n69 = global read "Global 1.vi" "Distance"() -> (w113:dbl)
          n70 = global read "Global 1.vi" "Positions"() -> (w112:dbl)
          n71 = call "FullAlign.vi"("Joystick 0"=w114, "Button"=TRUE, "Joystick 1"=w114, "Distance"=w113, "Angle"=w112) -> ("Right Motor"=w116:dbl, "Left Motor"=w115:dbl, "Not In Sight?"=w108:bool, "In Range?"=w111:bool)  [unwired: 7 in]
          n72 = case shown="True" w108 {
            selector: w108 -> [_ w133]
            tunnel: w116 -> [w118 _]
            tunnel: w115 -> [w117 _]
            tunnel: w110 -> [_ w131]
            frame False {
              n73 = call <vilib>:"WPI_MotorControlRefNum Registry Get.vi"("refnum name"="Drive R0") -> ("error out"=w124:errorcluster, "MotorControlDevRef"=w120:T5)  [unwired: 9 in]
              n74 = call <vilib>:"WPI_MotorControlRefNum Registry Get.vi"("refnum name"="Drive R1") -> ("error out"=w119:errorcluster, "MotorControlDevRef"=w122:T5)  [unwired: 9 in]
              n75 = call <vilib>:"WPI_MotorControlRefNum Registry Get.vi"("refnum name"="Drive L0") -> ("error out"=w125:errorcluster, "MotorControlDevRef"=w126:T5)  [unwired: 9 in]
              n76 = call <vilib>:"WPI_MotorControlRefNum Registry Get.vi"("refnum name"="Drive L1") -> ("error out"=w129:errorcluster, "MotorControlDevRef"=w128:T5)  [unwired: 9 in]
              n77 = call <vilib>:"WPI_MotorControlSetOutput.vi"("error in (no error)"=w124, "Output"=w118, "MotorControlDevRef"=w120) -> ()  [unwired: 6 in, 3 out]
              n78 = call <vilib>:"WPI_MotorControlSetOutput.vi"("error in (no error)"=w119, "Output"=w118, "MotorControlDevRef"=w122) -> ()  [unwired: 6 in, 3 out]
              n79 = call <vilib>:"WPI_MotorControlSetOutput.vi"("error in (no error)"=w125, "Output"=w117, "MotorControlDevRef"=w126) -> ()  [unwired: 6 in, 3 out]
              n80 = call <vilib>:"WPI_MotorControlSetOutput.vi"("error in (no error)"=w129, "Output"=w117, "MotorControlDevRef"=w128) -> ()  [unwired: 6 in, 3 out]
            }
            frame True {
              n81 = Not(x=w133) -> (.not. x?=w132:bool)
              n82 = call "Oscillate.vi"("Target In Sight?"=w132, "Effort"=w131) -> ()  [unwired: 10 in]
            }
          }
        }
      }
      frame "Turn", Default {
        n83 = flat-sequence {
          tunnel: w136 -> [w140]
          tunnel: w135 -> [w139]
          tunnel: w134 -> [w137]
          frame #0 {
            n84 = To Long Integer(number=w137) -> (32bit integer=w138:i32)
            n85 = Wait (ms)(milliseconds to wait=w139) -> ()  [unwired: 1 out]
            n86 = call "Turn.vi"("mode"=w138, "Effort"=w140) -> ()  [unwired: 10 in]
          }
          frame #1 {
            n87 = call "Turn.vi"("mode"=1, "Effort"=0.0) -> ()  [unwired: 10 in]
          }
        }
      }
      frame "Intake" {
        n88 = flat-sequence {
          tunnel: w144 -> [w146]
          tunnel: w143 -> [w145]
          frame #0 {
            n89 = Wait (ms)(milliseconds to wait=w145) -> ()  [unwired: 1 out]
            n90 = call "Intake.vi"("Effort"=w146) -> ()  [unwired: 11 in]
          }
          frame #1 {
            n91 = call "Intake.vi"("Effort"=0.0) -> ()  [unwired: 11 in]
          }
        }
      }
      frame "Test" {
      }
      frame "Gear0" {
        n92 = flat-sequence {
          tunnel: w148 -> [w152]
          frame #0 {
            n93 = To Unsigned Byte Integer(number=w152) -> (unsigned 8bit integer=w151:u8)
            n94 = Number To Boolean Array(number=w151) -> (Boolean array=w150:bool[])
            n95 = Index Array(array=w150) -> (element=w149:bool)  [unwired: 1 in]
            n96 = call "Gear.vi"("Gear0?"=w149) -> ()  [unwired: 11 in]
          }
        }
      }
      frame "Gear1" {
        n97 = flat-sequence {
          tunnel: w153 -> [w157]
          frame #0 {
            n98 = To Unsigned Byte Integer(number=w157) -> (unsigned 8bit integer=w156:u8)
            n99 = Number To Boolean Array(number=w156) -> (Boolean array=w155:bool[])
            n100 = Index Array(array=w155) -> (element=w154:bool)  [unwired: 1 in]
            n101 = call "Gear.vi"("Gear1?"=w154) -> ()  [unwired: 11 in]
          }
        }
      }
      frame "Index" {
        n102 = flat-sequence {
          tunnel: w159 -> [w160]
          tunnel: w158 -> [_]
          frame #0 {
            n103 = Wait (ms)(milliseconds to wait=w160) -> ()  [unwired: 1 out]
            n104 = call "Index.vi"("Shoot"=TRUE ("Override?"), "Output"=-1.0) -> ()  [unwired: 10 in]
          }
          frame #1 {
            n105 = call "Index.vi"("Shoot"=FALSE ("Override?"), "Output"=0.0) -> ()  [unwired: 10 in]
          }
        }
      }
      frame "Climb" {
        n106 = flat-sequence {
          tunnel: w166 -> [w168]
          tunnel: w165 -> [w167]
          frame #0 {
            n107 = call "Climb.vi"("Effort"=w168) -> ()  [unwired: 11 in]
            n108 = Wait (ms)(milliseconds to wait=w167) -> ()  [unwired: 1 out]
          }
          frame #1 {
            n109 = call "Climb.vi"("Effort"=0.0) -> ()  [unwired: 11 in]
          }
        }
      }
      frame "Drive Encoder Reset" {
        n110 = while {
          stop <- w170 stop-if-true
          n111 = call <vilib>:"WPI_MotorControlRefNum Registry Get.vi"("refnum name"="Drive L1") -> ("error out"=w180:errorcluster, "MotorControlDevRef"=w175:T5)  [unwired: 9 in]
          n112 = call <vilib>:"WPI_MotorControlRefNum Registry Get.vi"("refnum name"="Drive R1") -> ("error out"=w185:errorcluster, "MotorControlDevRef"=w184:T5)  [unwired: 9 in]
          n113 = call <vilib>:"WPI_MotorControlRefNum Registry Get.vi"("refnum name"="Drive L1") -> ("error out"=w187:errorcluster, "MotorControlDevRef"=w188:T5)  [unwired: 9 in]
          n114 = call <vilib>:"WPI_MotorControlRefNum Registry Get.vi"("refnum name"="Drive R1") -> ("error out"=w177:errorcluster, "MotorControlDevRef"=w176:T5)  [unwired: 9 in]
          n115 = call <vilib>:"WPI_CANTalonSRX_SetSensorPosition.vi"("error in (no error)"=w185, "New Sensor Position"=0.0, "CAN Talon SRX Ref"=w184) -> ()  [unwired: 7 in, 2 out]
          n116 = call <vilib>:"WPI_CANTalonSRX_SetSensorPosition.vi"("error in (no error)"=w187, "New Sensor Position"=0.0, "CAN Talon SRX Ref"=w188) -> ()  [unwired: 7 in, 2 out]
          n117 = call <vilib>:"WPI_CANTalonSRX_GetStatus.vi"("error in (no error)"=w180, "CAN Talon SRX Ref"=w175) -> ("Talon SRX Status"=w178:T9)  [unwired: 7 in, 2 out]
          n118 = Unbundle By Name(w178) -> ("Encoder Position"=w173:dbl)
          n119 = call <vilib>:"WPI_CANTalonSRX_GetStatus.vi"("error in (no error)"=w177, "CAN Talon SRX Ref"=w176) -> ("Talon SRX Status"=w179:T9)  [unwired: 7 in, 2 out]
          n120 = Unbundle By Name(w179) -> ("Encoder Position"=w174:dbl)
          n121 = Equal To 0?(x=w173) -> (x = 0?=w172:bool)
          n122 = Equal To 0?(x=w174) -> (x = 0?=w171:bool)
          n123 = And(x=w172, y=w171) -> (x .and. y?=w170:bool)
        }
      }
      frame "Gyro Reset" {
        n124 = while {
          stop <- w191 stop-if-true
          w194 = 0.3
          n125 = call <vilib>:"WPI_GyroRefNum Registry Get.vi"("refnum name"="Gyro") -> ("error out"=w196:errorcluster, "GyroDevRef"=w197:T10)  [unwired: 9 in]
          n126 = global read "Global 2.vi" "Gyro"() -> (w192:dbl)
          n127 = call <vilib>:"WPI_GyroReset.vi"("error in"=w196, "GyroDevRef"=w197) -> ()  [unwired: 8 in, 2 out]
          n128 = Negate(x=w194) -> (-x=w193:dbl)
          n129 = In Range and Coerce(upper limit=w194, x=w192, lower limit=w193) -> (In Range?=w191:bool)  [unwired: 1 out]
        }
      }
    }
  }
